vi "Frequency Offset Compensation (per Channel).vi"(10 "params":T2, 11 "sample in":T1) -> (1 "static frequency shift out":fxp<+/-,48,0>, 2 "output valid":bool, 3 "sample out":T1)   [LabVIEW 2020]
uses:
  <instrlib>/_niInstr/DSP/v1/Shared/Public/IQ Data.ctl
  <instrlib>/_niInstr/DSP/v1/FPGA/Public/Sub VIs/Frequency Shift/Frequency Shift - 1 spc.vi
  <vilib>/rvi/FXPMathLib/FxpInterpret/XNode/nifxpmath_Interpret.xnode
  <instrlib>/_niInstr/DSP/v1/XNodes/Public/Frequency Shift/niInstr DSP v1 Frequency Shift FPGA.xnode
  <instrlib>/_niInstr/DSP/v1/Shared/niInstr DSP v1 Shared.lvlib
  <instrlib>/_niInstr/DSP/v1/FPGA/niInstr DSP v1 FPGA.lvlib
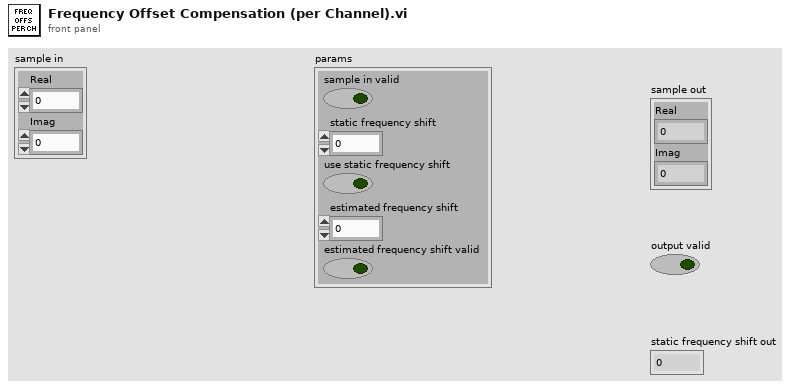
[diagram p1: front panel]
types:
  T1 = cluster{"Real":fxp<+/-,16,3>, "Imag":fxp<+/-,16,3>}
  T2 = cluster{"sample in valid":bool, "static frequency shift":fxp<+/-,48,0>, "use static frequency shift":bool, "estimated frequency shift":fxp<+/-,48,0>, "estimated frequency shift valid":bool}
  T3 = typedef "niInstr DSP v1 Shared.lvlib/IQ Data.ctl" = cluster{"I":fxp<+/-,18,1>, "Q":fxp<+/-,18,1>, "overflow":bool}
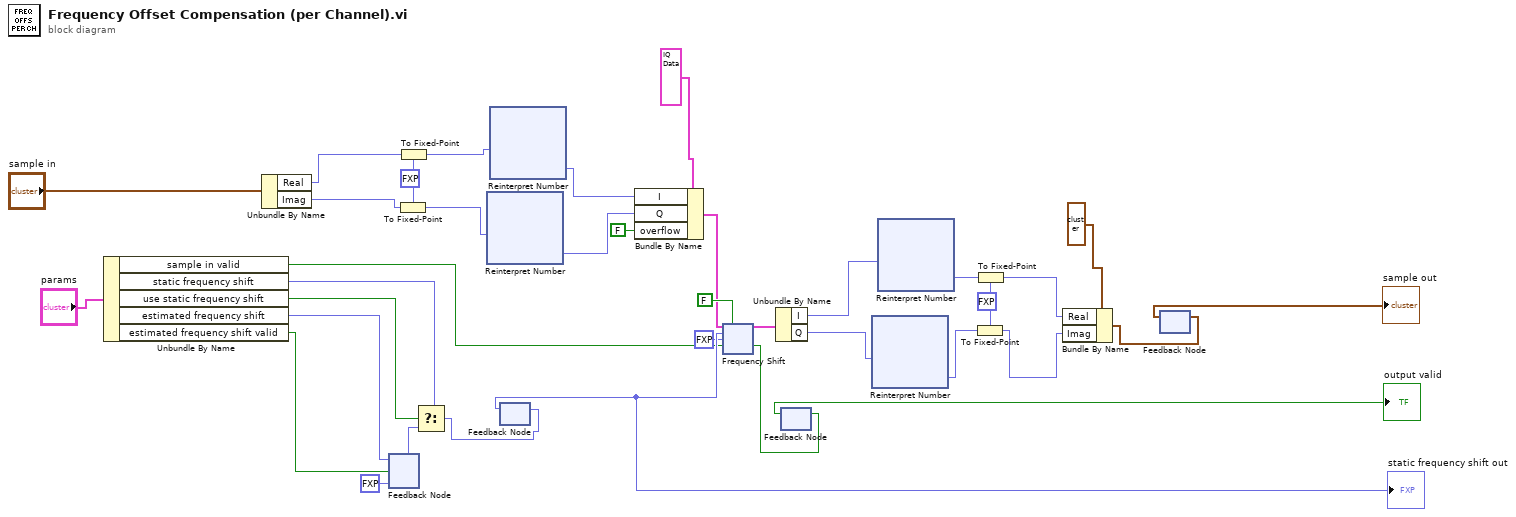
[diagram p0: block diagram]
diagram:
  w30 = fxp<+/-,16,3> 0.0 ("fixed-point type")
  w8 = fxp<+/-,18,3> 0.0 ("fixed-point type")
  n1 = Unbundle By Name("params") -> ("sample in valid"=w6:bool, "static frequency shift"=w5:fxp<+/-,48,0>, "use static frequency shift"=w4:bool, "estimated frequency shift"=w3:fxp<+/-,48,0>, "estimated frequency shift valid"=w2:bool)
  n2 = Unbundle By Name("sample in") -> ("Real"=w10:fxp<+/-,16,3>, "Imag"=w9:fxp<+/-,16,3>)
  n3 = feedback #1(fxp<+/-,48,0> 0.0 ("estimated frequency shift")) -> (w19:fxp<+/-,48,0>)
  n4 = feedback-in #1(w3, w2) -> ()
  n5 = To Fixed-Point(fixed-point type=w8, number=w9) -> (fixed-point=w12:fxp<+/-,18,3>)
  n6 = To Fixed-Point(fixed-point type=w8, number=w10) -> (fixed-point=w11:fxp<+/-,18,3>)
  n7 = Select(t=w5, s=w4, f=w19) -> (s? t:f=w21:fxp<+/-,48,0>)
  n8 = xnode "Reinterpret Number"("x"=w12) -> ("y"=w15:fxp<+/-,18,1>)
  n9 = xnode "Reinterpret Number"("x"=w11) -> ("y"=w14:fxp<+/-,18,1>)
  n10 = feedback #2() -> (w29:fxp<+/-,48,0>)  [unwired: 1 in]
  "static frequency shift out" <- w29
  n11 = feedback-in #2(w21) -> ()
  n12 = Bundle By Name(cluster=T3 {"I"=0.0, "Q"=0.0, "overflow"=FALSE} ("data in"), "I"=w14, "Q"=w15, "overflow"=FALSE) -> (w17:T3)
  n13 = xnode "Frequency Shift"("data in"=w17, "reset"=FALSE, "frequency shift"=w29, "phase"=fxp<+/-,21,0> 0.0, "input valid"=w6) -> ("data out"=w25:T3, "output valid"=w24:bool)  [unwired: 1 in, 1 out]
  n14 = Unbundle By Name(w25) -> ("I"=w26:fxp<+/-,18,1>, "Q"=w27:fxp<+/-,18,1>)
  n15 = feedback #3() -> (→"output valid":bool)  [unwired: 1 in]
  n16 = feedback-in #3(w24) -> ()
  n17 = xnode "Reinterpret Number"("x"=w27) -> ("y"=w31:fxp<+/-,18,3>)
  n18 = xnode "Reinterpret Number"("x"=w26) -> ("y"=w32:fxp<+/-,18,3>)
  n19 = To Fixed-Point(fixed-point type=w30, number=w31) -> (fixed-point=w34:fxp<+/-,16,3>)
  n20 = To Fixed-Point(fixed-point type=w30, number=w32) -> (fixed-point=w33:fxp<+/-,16,3>)
  n21 = Bundle By Name(cluster=T1 {"Real"=0.0, "Imag"=0.0} ("sample in"), "Real"=w33, "Imag"=w34) -> (w36:T1)
  n22 = feedback #4() -> (→"sample out":T1)  [unwired: 1 in]
  n23 = feedback-in #4(w36) -> ()
